vi "Read Integer Input File.vi"(11 "file path (dialog if empty)":path) -> (2 "input values":i64[](array[numeric]))   [LabVIEW 2021]
uses:
  <vilib>/Utility/file.llb/Read Delimited Spreadsheet (I64).vi
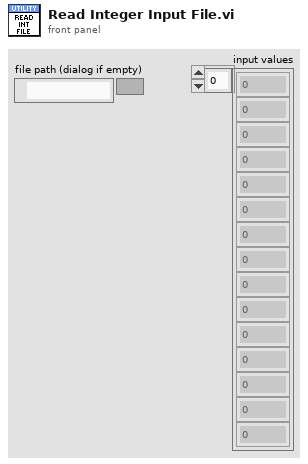
[diagram p1: front panel]
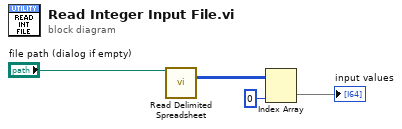
[diagram p0: block diagram]
diagram:
  n1 = call-poly <vilib>:"Read Delimited Spreadsheet.vi"("file path (dialog if empty)"="file path (dialog if empty)") -> ("all rows"=w3:i64[][])  [unwired: 9 in, 5 out]
  n2 = Index Array(array=w3, index (col)=0 ("disabled index (col)")) -> (element=→"input values":i64[])  [unwired: 1 in]
